vi "Array Dim(s) from TD.vi"(8 "error in (no error)":errorcluster, 10 "Array Type Descriptor":refnum<class "Array.lvclass">) -> (0 "error out":errorcluster, 2 "N dims":u32)   [LabVIEW 2020, in "lvdata.lvlib" / "type_descriptor.lvlib" / "Array.lvclass"]
doc: "Returns the number dimensions described by array type descriptor input."
uses:
  ArrayTD/Array.lvclass
  C:/projects/OpenG-Variant-Data-Library/source/library/LVData/Type Descriptor/TypeDescriptor.lvclass
  Bytes/Bytes.lvclass/Bytes.ctl
  get_num_elements.vi/b3898c1b-5169-4cb1-894b-457c92b4a1c3.vi
  get_num_elements.vi/b3898c1b-5169-4cb1-894b-457c92b4a1c3.vi/81433c74-ee36-47cf-a886-10c868675b30.vi
  get_num_elements.vi/b3898c1b-5169-4cb1-894b-457c92b4a1c3.vi/d8d9ff34-2c15-4edb-a5ad-7260f11560db.vi
  Bytes/read.vi
  Bytes/to_data.vi
  Bytes/from_byte_array.vi
  TypeDescriptor.lvclass
  C:/projects/OpenG-Variant-Data-Library/source/library/Bytes/Bytes.lvclass
  Bytes/Bytes.lvclass
panel:
  # "[OpenG VI Tags] ***Do Not Remove***"
  # "Array Dim(s) from TD.vi\n\nReturns the number dimensions described by array type descriptor input.\n\nPlease visit http://www.OpenG.org to learn about the\nOpen Source LabVIEW software movement.\n\nNOTICE -- YOU MUST LEAVE THIS NOTICE IN PLACE.  PER THE TERMS OF THE LICENSE BELOW, YOU MAY SUBLICENSE THIS SOFTWARE \nIN ANY WAY THAT DOES NOT CONFLICT WITH THIS LICENSE.\n\n### BSD License (http://www.opensource.org/licenses/bsd-license.php) Begin ###\n \nCopyright (c) 2002, Jean-Pierre Drolet <drolet_jp@hotmail.com>\nCopyright (c) 2002-2006, Jim Kring <jim@jimkring.com>\n\nAll rights reserved.\n\nRedistribution and use in source and binary forms, with or without modification, are permitted provided that the following conditions are met:\n\n    * Redistributions of source code must retain the above copyright notice, this list of conditions and the following disclaimer.\n    * Redistributions in binary form must reproduce the above copyright notice, this list of conditions and the following disclaimer in the \n       documentation and/or other materials provided with the distribution.\n    * Neither the name of SciWare, James Kring, Inc., nor the names of its contributors may be used to endorse or promote products derived \n       from this software without specific prior written permission.\n\nTHIS SOFTWARE IS PROVIDED BY THE COPYRIGHT HOLDERS AND CONTRIBUTORS \"AS IS\" AND ANY EXPRESS OR IMPLIED WARRANTIES, \nINCLUDING, BUT NOT LIMITED TO, THE IMPLIED WARRANTIES OF MERCHANTABILITY AND FITNESS FOR A PARTICULAR PURPOSE ARE \nDISCLAIMED. IN NO EVENT SHALL THE COPYRIGHT OWNER OR CONTRIBUTORS BE LIABLE FOR ANY DIRECT, INDIRECT, INCIDENTAL,\n SPECIAL, EXEMPLARY, OR CONSEQUENTIAL DAMAGES (INCLUDING, BUT NOT LIMITED TO, PROCUREMENT OF SUBSTITUTE GOODS OR \nSERVICES; LOSS OF USE, DATA, OR PROFITS; OR BUSINESS INTERRUPTION) HOWEVER CAUSED AND ON ANY THEORY OF LIABILITY, \nWHETHER IN CONTRACT, STRICT LIABILITY, OR TORT (INCLUDING NEGLIGENCE OR OTHERWISE) ARISING IN ANY WAY OUT OF THE USE \nOF THIS SOFTWARE, EVEN IF ADVISED OF THE POSSIBILITY OF SUCH DAMAGE.\n\n### BSD License End ###"
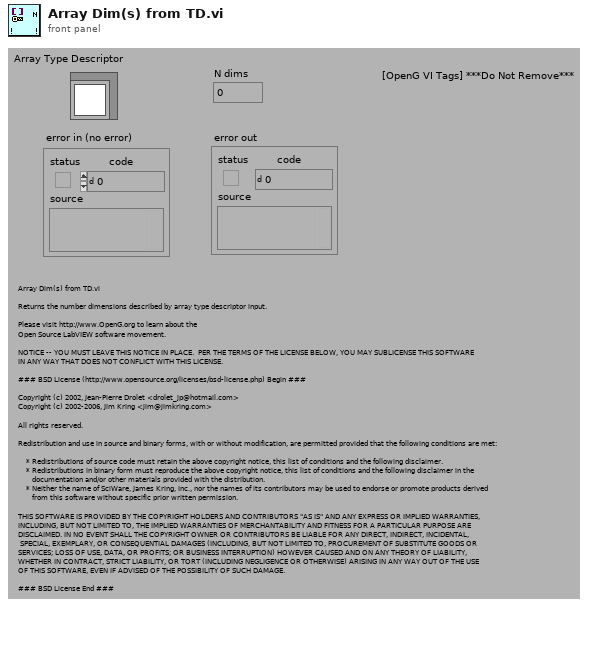
[diagram p1: front panel]
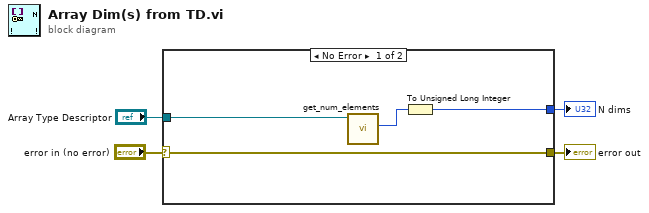
[diagram p0: block diagram]
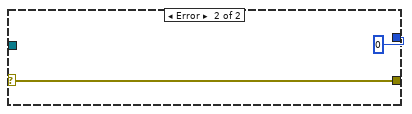
[diagram p2: hidden frame]
diagram:
  n1 = case shown="No Error" "error in (no error)" {
    selector: "error in (no error)" -> [w6 w10]
    tunnel: [w8 u32 0] -> w4
    tunnel: "Array Type Descriptor" -> [w7 _]
    tunnel: [w6 w10] -> w2
    frame No Error {
      n2 = call "get_num_elements.vi"("TypeDescriptor"=w7) -> ("num_element"=w5:i32)  [unwired: 9 in, 1 out]
      n3 = To Unsigned Long Integer(number=w5) -> (unsigned 32bit integer=w8:u32)
    }
    frame Error {
    }
  }
  "N dims" <- w4
  "error out" <- w2
